vi "injector magnet.vi"() -> ()   [LabVIEW 2016]
uses:
  Controls/Isotope type.ctl
  Controls/Injector Field Settings.ctl
  Top level/features/field/Injector global.vi
panel:
  in  "Rare Field":dbl(slide) scale=0.3..0.5
  in  "Stable 1 Field":dbl format="%#_7g"
  in  "Stable 2 Field":dbl format="%#_7g"
  out "Injector Field Setpoint":dbl
  in  "Isotope":T1
  in  "reset injector":bool
  out "Measured Injector Field":dbl
  in  "Scale":bool
  in  "stop":bool
  out "Waveform Chart":dbl(graph)
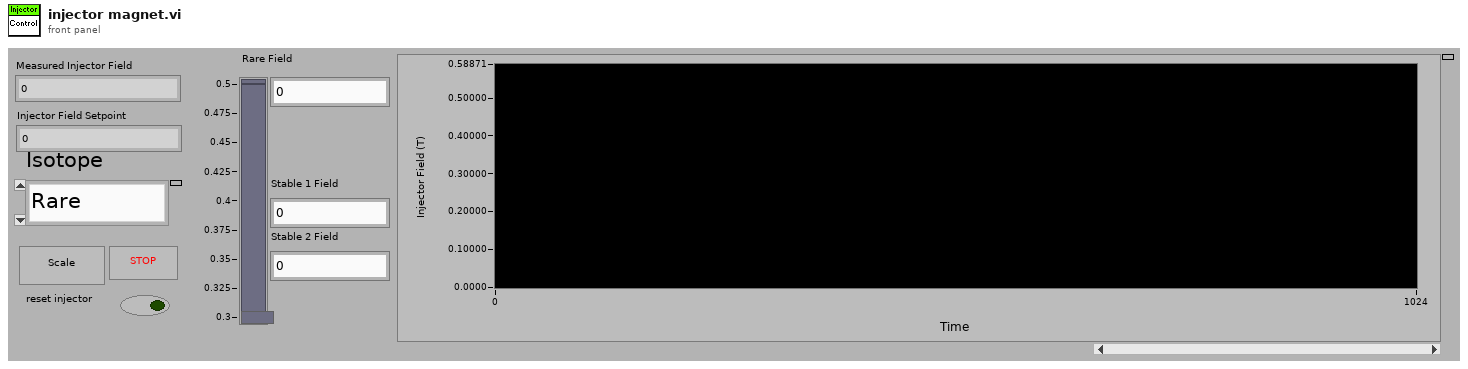
[diagram p1: front panel]
types:
  T1 = typedef "Isotope type.ctl" = enum16{"Rare", "Stable 1", "Stable 2"}
  T2 = typedef "Injector Field Settings.ctl" = cluster{"Stable 1":dbl, "Rare":dbl, "Stable 2":dbl}
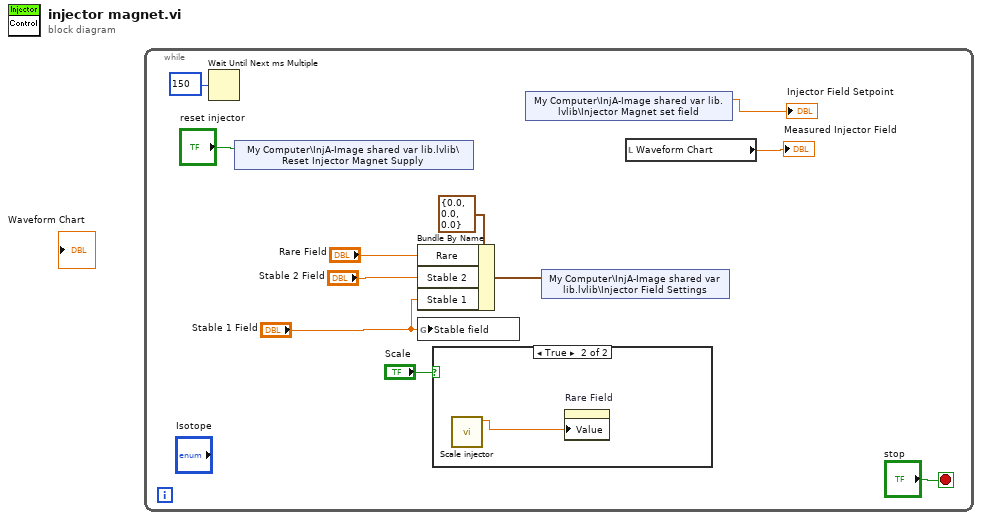
[diagram p0: block diagram]
diagram:
  n1 = while {
    stop <- "stop" stop-if-true
    n2 = Wait Until Next ms Multiple(millisecond multiple=u32 150) -> ()  [unwired: 1 out]
    n3 = shared-variable "My Computer\\InjA-Image shared var lib.lvlib\\Reset Injector Magnet Supply"("reset injector") -> ()  [unwired: 1 in, 1 out]
    n4 = Bundle By Name(cluster=T2 {"Stable 1"=0.0, "Rare"=0.0, "Stable 2"=0.0} ("Injector Field Settings"), "Rare"="Rare Field", "Stable 2"="Stable 2 Field", "Stable 1"="Stable 1 Field") -> (w4:T2)
    n5 = global write "Injector global.vi" "Stable field"("Stable 1 Field") -> ()
    n6 = case shown="True" "Scale" {
      frame False {
      }
      frame True {
        n7 = call "Scale injector.vi"() -> ("Rare Field"=w12:dbl)  [unwired: 11 out]
        n8 = property on="Rare Field" class="Slide (strict)"("Value"=w12) -> ()  [unwired: 2 in, 2 out]
      }
    }
    n9 = shared-variable "My Computer\\InjA-Image shared var lib.lvlib\\Injector Magnet set field"() -> (→"Injector Field Setpoint":dbl)  [unwired: 1 in, 1 out]
    n10 = shared-variable "My Computer\\InjA-Image shared var lib.lvlib\\Injector Field Settings"(w4) -> ()  [unwired: 1 in, 1 out]
    n11 = local read "Waveform Chart"() -> (→"Measured Injector Field":dbl)
  }
